vi "Create.vi"(5 "VolatusAPI":refnum<class "VolatusAPI.lvclass">, 7 "Variables":refnum<class "Variables.lvclass">, 10 "error in (no error)":errorcluster, 11 "F String":string) -> (2 "error out":errorcluster, 3 "Format String out":refnum<class "Format String.lvclass">)   [LabVIEW 2020, in "VolatusSeq.lvlib" / "Format String.lvclass"]
uses:
  Format String.lvclass
  Variables/Variables.lvclass
  Volatus/VolatusAPI/VolatusAPI.lvclass
  Format String.lvclass/Format String.ctl
  Condition Value/Condition Value.lvclass
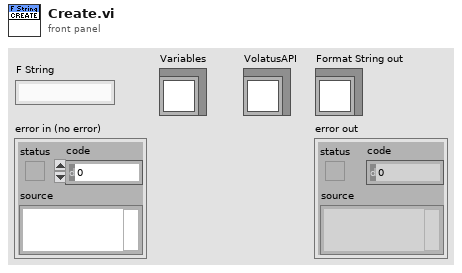
[diagram p1: front panel]
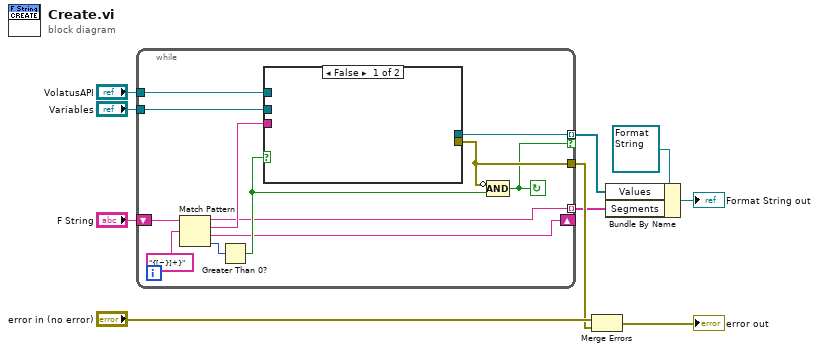
[diagram p0: block diagram]
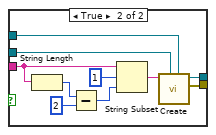
[diagram p2: hidden frame]
diagram:
  n1 = while {
    shift-right: [w12] -> _
    shift-left: "F String" -> [w20]
    tunnel: "VolatusAPI" -> [w16]
    tunnel: "Variables" -> [w17]
    tunnel: [w14] -> w1 mode=indexing if=w13
    tunnel: [w22] -> w4
    tunnel: [w11] -> w2 mode=indexing
    stop <- w13 continue-if-true
    n2 = Match Pattern(string=w20, regular expression="{[~}]+}") -> (before substring=w11:string, match substring=w18:string, after substring=w12:string, offset past match=w19:i32)  [unwired: 1 in]
    n3 = Greater Than 0?(x=w19) -> (x > 0?=w15:bool)
    n4 = case shown="False" w15 {
      tunnel: w18 -> [_ w30]
      tunnel: w17 -> [_ w26]
      tunnel: w16 -> [_ w25]
      tunnel: [_ w24] -> w14
      tunnel: [_ w23] -> w22
      frame False {
      }
      frame True {
        n5 = String Length(string=w30) -> (length=w32:i32)
        n6 = Subtract(x=w32, y=2) -> (x-y=w29:i32)
        n7 = String Subset(string=w30, offset (0)=1, length (rest)=w29) -> (substring=w27:string)
        n8 = call "Create.vi"("VolatusAPI"=w25, "Variables"=w26, "Source Name"=w27) -> ("error out"=w23:errorcluster, "Condition Value out"=w24:refnum<class "Condition Value.lvclass">)  [unwired: 7 in]
      }
    }
    n9 = Compound Arithmetic op=AND(invert w22, w15) -> (w13:bool)
  }
  n10 = Merge Errors("error in (no error)", w4) -> (→"error out":errorcluster)
  n11 = Bundle By Name(cluster=refnum<class "Format String.lvclass"> refnum ("Format String in"), "Values"=w1, "Segments"=w2) -> (→"Format String out":refnum<class "Format String.lvclass">)
